vi "DEV Read User Data.vi"(7 "DataLen":i32, 9 "pReadData":string, 10 "OffsetAddr":i32, 11 "DevHandle":i32) -> (1 "pReadData out":string, 3 "function return":u8)   [LabVIEW 2010, in "usb_device.lvlib"]
doc: "unsigned char WINAPI DEV_ReadUserData(int DevHandle,int OffsetAddr,unsigned char *pReadData,int DataLen);"
uses:
  usb_device.lvlib
  USB2XXX/trunk/USB2XXX/USB2XXX/vs2019/Release/USB2XXX.dll
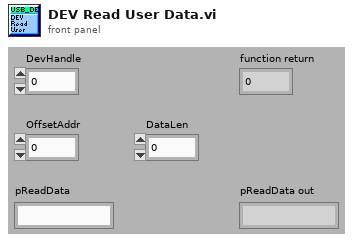
[diagram p1: front panel]
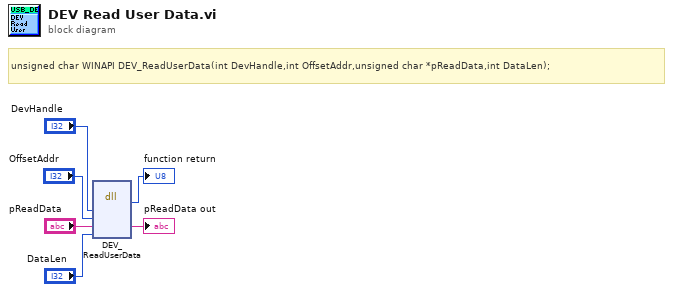
[diagram p0: block diagram]
diagram:
  # "unsigned char WINAPI DEV_ReadUserData(int DevHandle,int OffsetAddr,unsigned char *pReadData,int DataLen);"
  n1 = dll-call lib="E:/Projects/USB2XXX/trunk/USB2XXX/USB2XXX/vs2019/Release/USB2XXX.*" fn="DEV_ReadUserData"("DevHandle"="DevHandle", "OffsetAddr"="OffsetAddr", "pReadData"="pReadData", "DataLen"="DataLen") -> (→"function return":u8, "pReadData"=→"pReadData out":string)  [unwired: 6 in, 2 out]
